vi "解析原值.vi"(8 "原值":string, 11 "补充信息":string[](array[string])) -> (3 "参数":string[](array[string]))   [LabVIEW 2018]
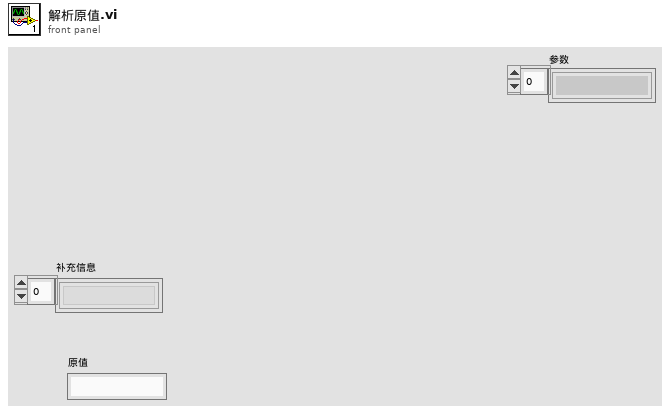
[diagram p1: front panel]
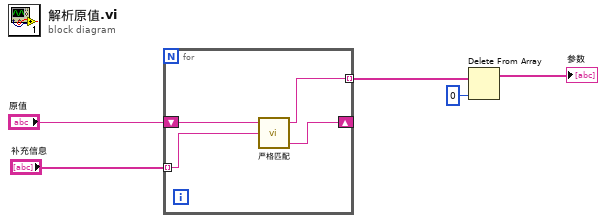
[diagram p0: block diagram]
diagram:
  n1 = for {
    tunnel: "补充信息" -> [w8] mode=indexing
    shift-right: [w6] -> _
    shift-left: "原值" -> [w9]
    tunnel: [w7] -> w3 mode=indexing
    n2 = call "严格匹配.vi"("搜索字符串"=w8, "输入字符串"=w9) -> ("之后"=w6:string, "之前"=w7:string)  [unwired: 1 in, 1 out]
  }
  n3 = Delete From Array(array=w3, index=0 ("索引")) -> (array with subset deleted=→"参数":string[])  [unwired: 1 in, 1 out]
